vi "按工单数量查询.vi"(5 "Timeout":i32, 6 "MO":string, 7 "DBSet":T1, 8 "test result":bool, 9 "PN":string) -> (2 "当前数量":string)   [LabVIEW 2011]
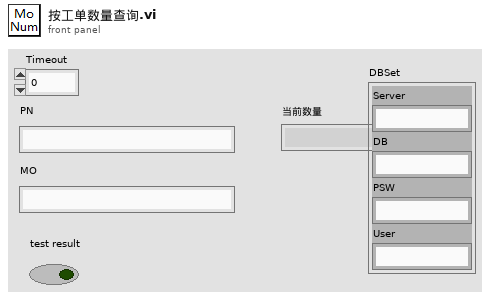
[diagram p1: front panel]
types:
  T1 = cluster{"Server":string, "DB":string, "PSW":string, "User":string}
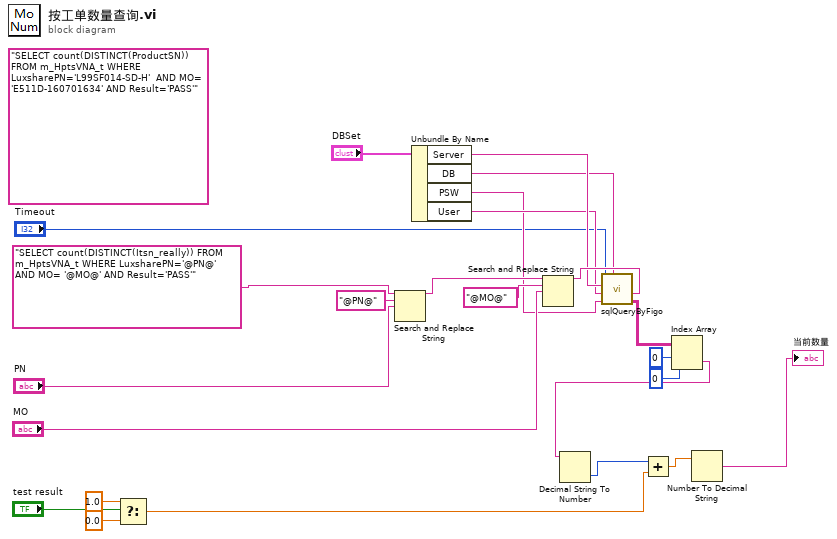
[diagram p0: block diagram]
diagram:
  (unwired) "SELECT count(DISTINCT(ProductSN)) FROM m_HptsVNA_t WHERE LuxsharePN='L99SF014-SD-H'  AND MO= 'E511D-160701634' AND Result='PASS'" ("SQL")
  n1 = Select(t=1.0, s="test result", f=0.0) -> (s? t:f=w9:dbl)
  n2 = Search and Replace String(input string="SELECT count(DISTINCT(Itsn_really)) FROM m_HptsVNA_t WHERE LuxsharePN='@PN@'  AND MO= '@MO@' AND Result='PASS'" ("SQL"), search string="@PN@" ("搜索字符串"), replace string="PN") -> (result string=w21:string)  [unwired: 5 in, 3 out]
  n3 = Unbundle By Name("DBSet") -> ("Server"=w5:string, "DB"=w2:string, "PSW"=w3:string, "User"=w4:string)
  n4 = Search and Replace String(input string=w21, search string="@MO@" ("搜索字符串"), replace string="MO") -> (result string=w18:string)  [unwired: 5 in, 3 out]
  n5 = call "sqlQueryByFigo.vi"("SQL"=w18, "DATABASE"=w2, "password"=w3, "user id"=w4, "Server"=w5, "Timeout"="Timeout") -> ("查询数据"=w17:string[][])  [unwired: 4 in, 1 out]
  n6 = Index Array(array=w17, index (row)=0 ("索引 (行)"), index (col)=0 ("禁用的索引 (列)")) -> (element=w11:string)
  n7 = Decimal String To Number(string=w11) -> (number=w10:i32)  [unwired: 2 in, 1 out]
  n8 = Add(x=w10, y=w9) -> (x+y=w8:dbl)
  n9 = Number To Decimal String(number=w8) -> (decimal integer string=→"当前数量":string)  [unwired: 1 in]
